vi "OPC UA.vi"() -> ()   [LabVIEW 2022 SP3]
uses:
  <vilib>/OPCUA/controls/Data Type.ctl
  <vilib>/OPCUA/NI OPC UA Server.lvlib
panel:
  out "Environment Temperature node ID":string
  out "error out":errorcluster
  in  "error in":errorcluster
  out "Setpoint Temperature node ID":string
  out "Folder node ID":string
  out "Control Voltage node ID":string
  out "Air Heter Temperature node ID":string
  out "Server Endpoint URL":string
  in  "Stop Button":bool
  # "OPC UA Server"
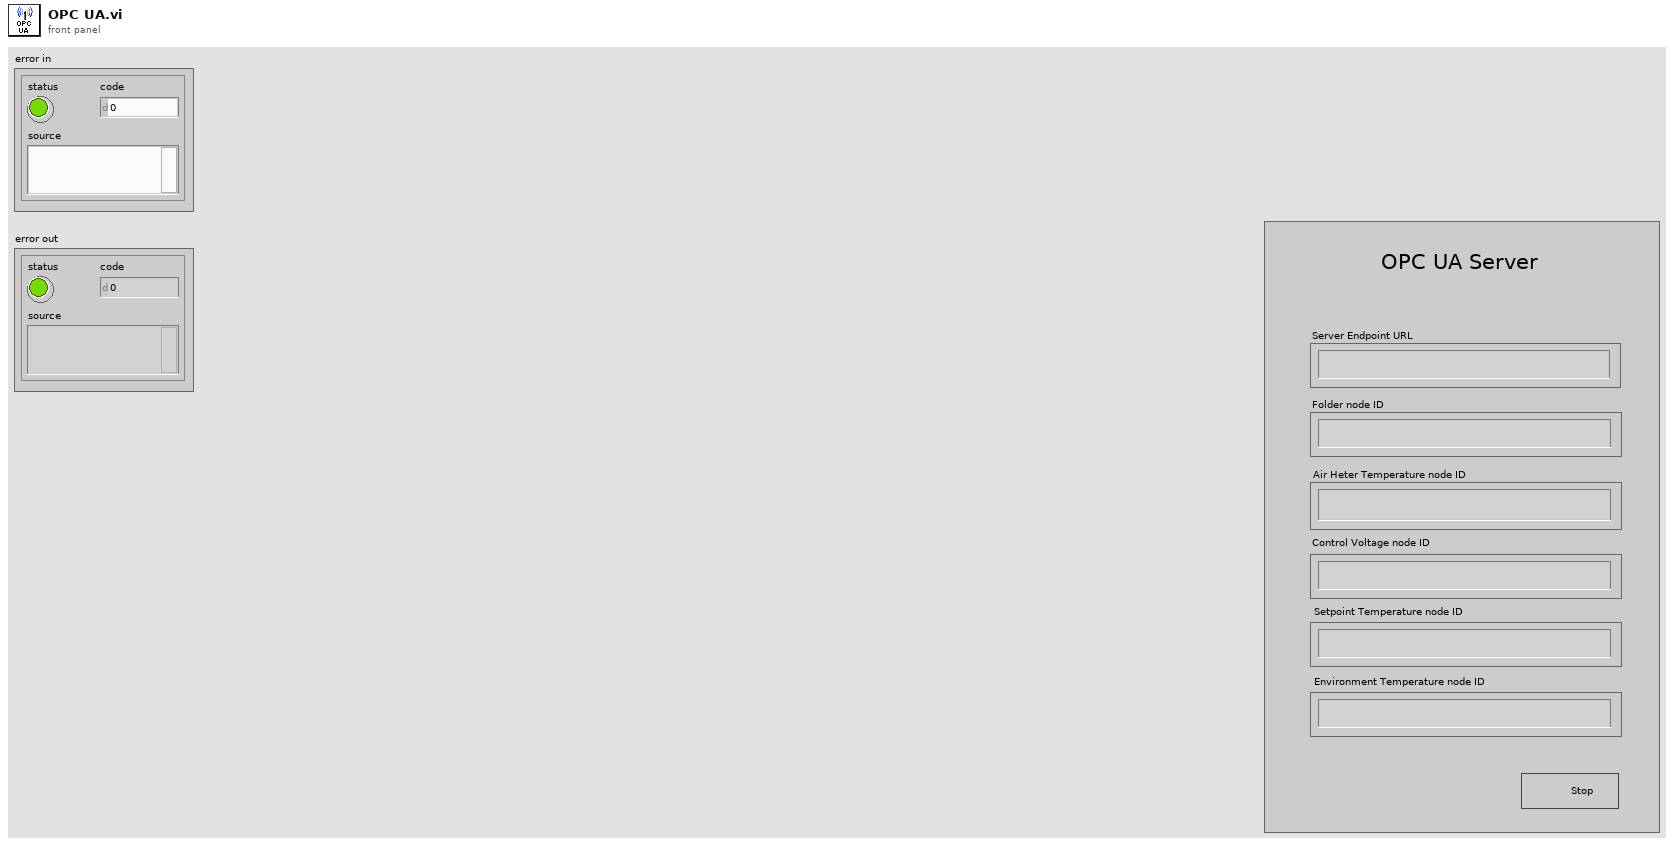
[diagram p1: front panel]
types:
  T1 = typedef "OPC UA Server Refnum.ctl" = refnum<k21>
  T2 = typedef "NodeId.ctl" = string
  T3 = typedef "Data Type.ctl" = u16
  T4 = cluster{"name":string, "data type":T3, "access level":u16, "description":string}
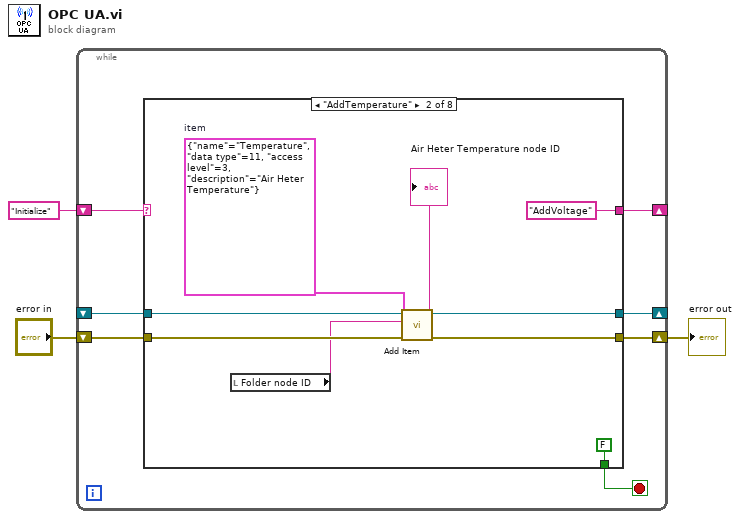
[diagram p0: block diagram]
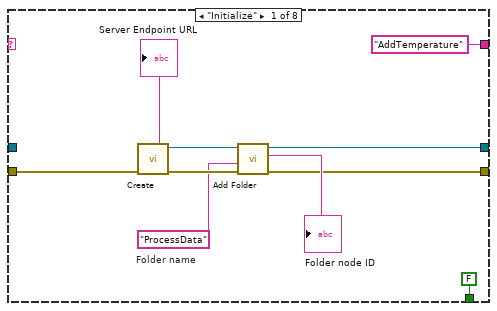
[diagram p2: hidden frame]
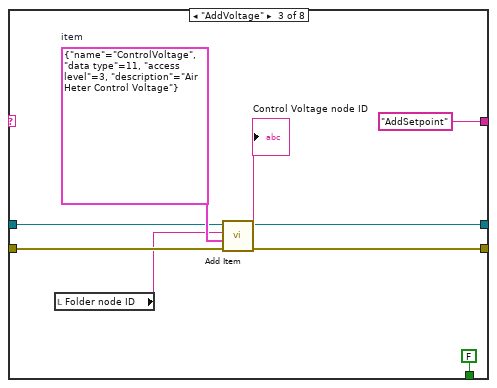
[diagram p3: hidden frame]
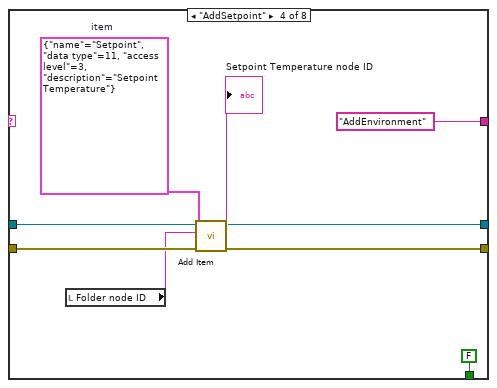
[diagram p4: hidden frame]
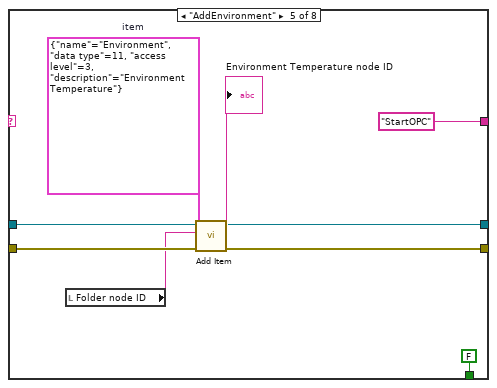
[diagram p5: hidden frame]
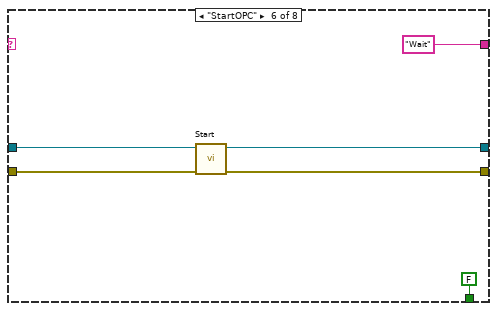
[diagram p6: hidden frame]
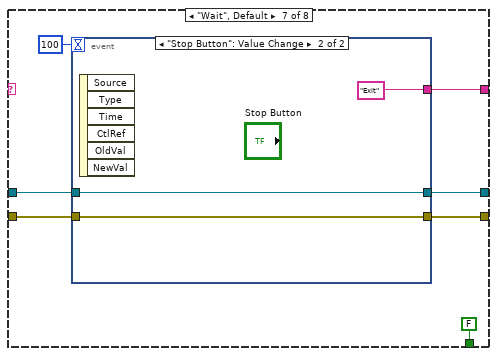
[diagram p7: hidden frame]
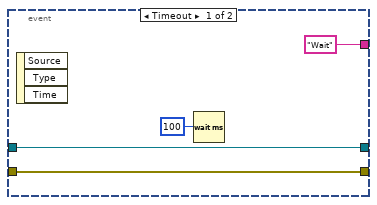
[diagram p8: hidden frame]
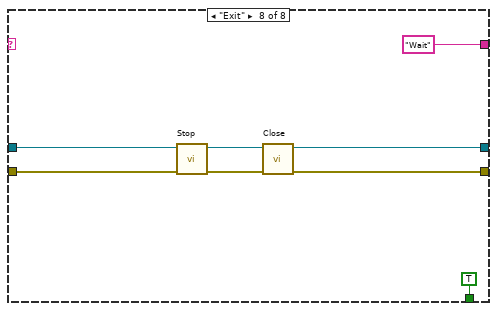
[diagram p9: hidden frame]
diagram:
  n1 = while {
    shift-right: [w9] -> _
    shift-left: "Initialize" -> [w10]
    shift-right: [w4] -> w1
    shift-left: "error in" -> [w7]
    shift-right: [w5] -> _
    shift-left: _ -> [w6]
    stop <- w8 stop-if-true
    n2 = case shown="\"AddTemperature\"" w10 {
      tunnel: ["AddTemperature" "AddVoltage" "AddSetpoint" "AddEnvironment" "StartOPC" "Wait" w68 "Wait"] -> w9
      tunnel: [FALSE FALSE FALSE FALSE FALSE FALSE FALSE TRUE] -> w8
      tunnel: w7 -> [w13 w26 w35 w43 w52 w60 w66 w80]
      tunnel: w6 -> [_ w25 w34 w42 w51 w58 w65 w79]
      tunnel: [w12 w24 w33 w41 w50 w59 w64 w78] -> w5
      tunnel: [w11 w21 w30 w39 w48 w57 w63 w77] -> w4
      frame "Initialize" {
        w17 = "ProcessData"  # Folder name
        n3 = call <vilib>:"Create.vi"("error in (no error)"=w13) -> ("error out"=w18:errorcluster, "server endpoint URL"=→"Server Endpoint URL":string, "OPC UA server refnum out"=w19:T1)  [unwired: 8 in]
        n4 = call <vilib>:"Add Folder.vi"("error in (no error)"=w18, "folder name"=w17, "OPC UA server refnum in"=w19) -> ("error out"=w11:errorcluster, "folder node ID"=→"Folder node ID":T2, "OPC UA server refnum out"=w12:T1)  [unwired: 5 in]
      }
      frame "AddTemperature" {
        w28 = T4 {"name"="Temperature", "data type"=11, "access level"=3, "description"="Air Heter Temperature"}  # item
        n5 = local read "Folder node ID"() -> (w22:string)
        n6 = call <vilib>:"Add Item.vi"("error in (no error)"=w26, "item"=w28, "parent folder node ID"=w22, "OPC UA server refnum in"=w25) -> ("error out"=w21:errorcluster, "item node ID"=→"Air Heter Temperature node ID":T2, "OPC UA server refnum out"=w24:T1)  [unwired: 3 in, 1 out]
      }
      frame "AddVoltage" {
        w37 = T4 {"name"="ControlVoltage", "data type"=11, "access level"=3, "description"="Air Heter Control Voltage"}  # item
        n7 = local read "Folder node ID"() -> (w32:string)
        n8 = call <vilib>:"Add Item.vi"("error in (no error)"=w35, "item"=w37, "parent folder node ID"=w32, "OPC UA server refnum in"=w34) -> ("error out"=w30:errorcluster, "item node ID"=→"Control Voltage node ID":T2, "OPC UA server refnum out"=w33:T1)  [unwired: 3 in, 1 out]
      }
      frame "AddSetpoint" {
        w46 = T4 {"name"="Setpoint", "data type"=11, "access level"=3, "description"="Setpoint Temperature"}  # item
        n9 = local read "Folder node ID"() -> (w40:string)
        n10 = call <vilib>:"Add Item.vi"("error in (no error)"=w43, "item"=w46, "parent folder node ID"=w40, "OPC UA server refnum in"=w42) -> ("error out"=w39:errorcluster, "item node ID"=→"Setpoint Temperature node ID":T2, "OPC UA server refnum out"=w41:T1)  [unwired: 3 in, 1 out]
      }
      frame "AddEnvironment" {
        w55 = T4 {"name"="Environment", "data type"=11, "access level"=3, "description"="Environment Temperature"}  # item
        n11 = local read "Folder node ID"() -> (w49:string)
        n12 = call <vilib>:"Add Item.vi"("error in (no error)"=w52, "item"=w55, "parent folder node ID"=w49, "OPC UA server refnum in"=w51) -> ("error out"=w48:errorcluster, "item node ID"=→"Environment Temperature node ID":T2, "OPC UA server refnum out"=w50:T1)  [unwired: 3 in, 1 out]
      }
      frame "StartOPC" {
        n13 = call <vilib>:"Start.vi"("error in (no error)"=w60, "OPC UA server refnum in"=w58) -> ("error out"=w57:errorcluster, "OPC UA server refnum out"=w59:T1)  [unwired: 7 in, 1 out]
      }
      frame "Wait", Default {
        n14 = event shown="[1] \"Stop Button\": Value Change" {
          selector: _ -> [_ _]
          dyn-events: _ -> [_ _]
          timeout: 100 -> [_ _]
          tunnel: ["Wait" "Exit"] -> w68
          tunnel: [w71 w75] -> w63
          tunnel: w66 -> [w71 w75]
          tunnel: [w70 w74] -> w64
          tunnel: w65 -> [w70 w74]
          event Timeout {
            n15 = event-data() -> ()  [unwired: 1 in, 3 out]
            n16 = Wait (ms)(milliseconds to wait=u32 100) -> ()  [unwired: 1 out]
          }
          event "Stop Button": Value Change {
            n17 = event-data() -> ()  [unwired: 1 in, 6 out]
          }
        }
      }
      frame "Exit" {
        n18 = call <vilib>:"Stop.vi"("error in (no error)"=w80, "OPC UA server refnum in"=w79) -> ("error out"=w82:errorcluster, "OPC UA server refnum out"=w78:T1)  [unwired: 8 in]
        n19 = call <vilib>:"Close.vi"("error in (no error)"=w82, "OPC UA server refnum in"=w78) -> ("error out"=w77:errorcluster)  [unwired: 9 in]
      }
    }
  }
  "error out" <- w1
